vi "Generate Grid Position.vi"(0 "Image Size":i32=4, 5 "Edge Size":i32=4, 7 "# of Steps":i32=4, 9 "init x pos":dbl format="%#_13g", 11 "init y pos":dbl format="%#_13g", 12 "Pixel Size":dbl=5.0) -> (4 "x grid pos":dbl[](array[numeric]), 6 "y grid pos":dbl[](array[numeric]))   [LabVIEW 2016]
panel:
  out "XY Graph":cluster{dbl[], dbl[]}(graph)
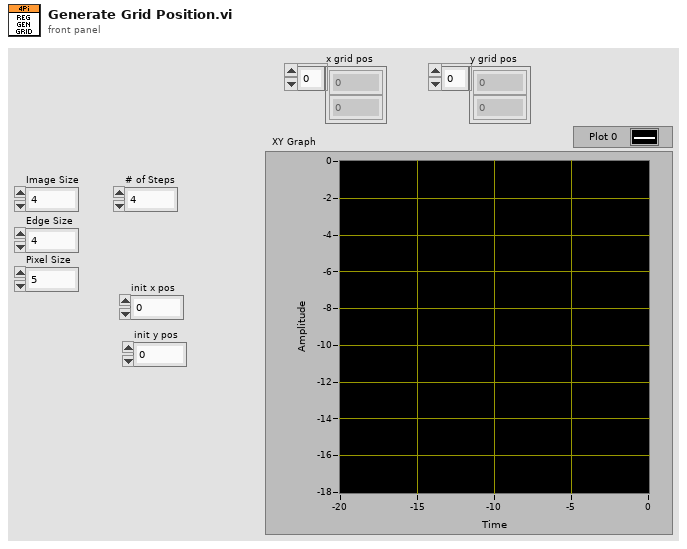
[diagram p1: front panel]
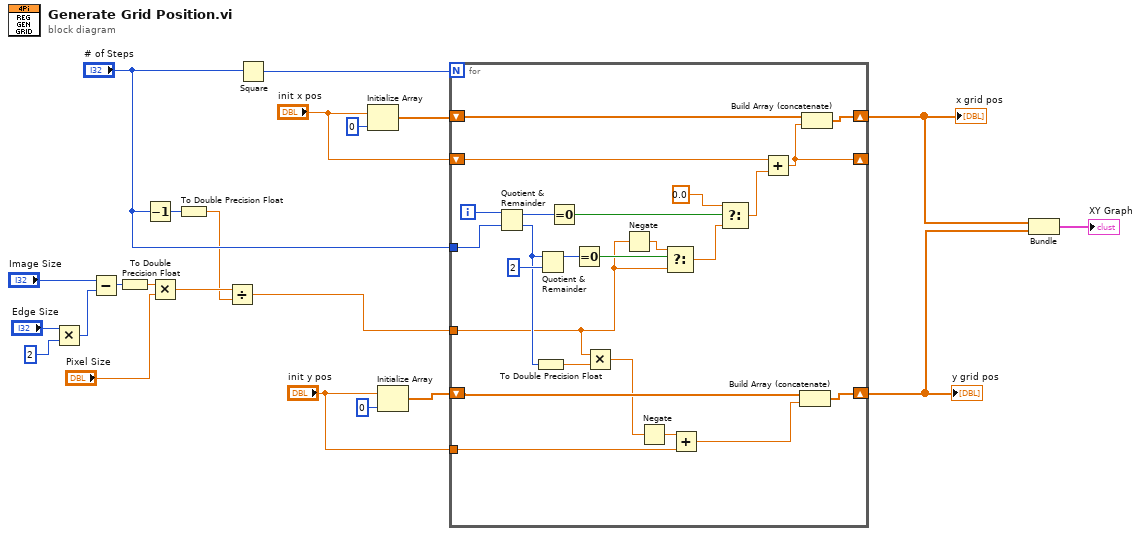
[diagram p0: block diagram]
diagram:
  n1 = Multiply(x="Edge Size", y=2) -> (x*y=w9:i32)
  n2 = Subtract(x="Image Size", y=w9) -> (x-y=w7:i32)
  n3 = To Double Precision Float(number=w7) -> (double precision float=w8:dbl)
  n4 = Decrement(x="# of Steps") -> (x-1=w3:i32)
  n5 = Multiply(x=w8, y="Pixel Size") -> (x*y=w5:dbl)
  n6 = To Double Precision Float(number=w3) -> (double precision float=w2:dbl)
  n7 = Divide(x=w5, y=w2) -> (x/y=w1:dbl)
  n8 = Square(x="# of Steps") -> (x^2=w19:i32)
  n9 = Initialize Array("init x pos", 0 ("dimension size")) -> (w20:dbl[])
  n10 = Initialize Array("init y pos", 0 ("dimension size")) -> (w17:dbl[])
  n11 = for {
    N: w19 -> [_]
    shift-right: [w44] -> _
    shift-left: "init x pos" -> [w46]
    shift-right: [w43] -> w16
    shift-left: w20 -> [w45]
    tunnel: "# of Steps" -> [w35]
    tunnel: w1 -> [w25]
    shift-right: [w31] -> w15
    shift-left: w17 -> [w33]
    tunnel: "init y pos" -> [w27]
    i -> [w42]
    n12 = Quotient & Remainder(x=w42, y=w35) -> (x-y*floor(x/y)=w41:i32, floor(x/y)=w29:i32)
    n13 = To Double Precision Float(number=w29) -> (double precision float=w28:dbl)
    n14 = Quotient & Remainder(x=w29, y=2) -> (x-y*floor(x/y)=w38:i32)  [unwired: 1 out]
    n15 = Equal To 0?(x=w41) -> (x = 0?=w30:bool)
    n16 = Equal To 0?(x=w38) -> (x = 0?=w34:bool)
    n17 = Multiply(x=w25, y=w28) -> (x*y=w24:dbl)
    n18 = Negate(x=w25) -> (-x=w26:dbl)
    n19 = Negate(x=w24) -> (-x=w23:dbl)
    n20 = Select(t=w26, s=w34, f=w25) -> (s? t:f=w37:dbl)
    n21 = Add(x=w23, y=w27) -> (x+y=w32:dbl)
    n22 = Select(t=0.0, s=w30, f=w37) -> (s? t:f=w36:dbl)
    n23 = Add(x=w46, y=w36) -> (x+y=w44:dbl)
    n24 = Build Array (concatenate)(w33, w32) -> (w31:dbl[])
    n25 = Build Array (concatenate)(w45, w44) -> (w43:dbl[])
  }
  "x grid pos" <- w16
  "y grid pos" <- w15
  n26 = Bundle(w16, w15) -> (→"XY Graph":cluster{dbl[], dbl[]})  [unwired: 1 in]
